vi "VisionMain_7.vi"(0 "Image In":T1, 7 "error in":errorcluster) -> (20 "Image Out":T1, 21 "Calibrated Centroid (PegLocation)":cluster{"X Centroid":sgl, "Y Centroid":sgl} {"Y Centroid" format="%.2f"; "X Centroid" format="%.2f"}, 22 "Particle Measurements (Real-World) (BoxValues)":dbl[][](array[numeric]) format="%.2f", 27 "error out":errorcluster)   [LabVIEW 2016]
uses:
  <vilib>/vision/Image Controls.llb/IMAQ Image.ctl
  <vilib>/vision/NI_Vision_Development_Module.lvlib
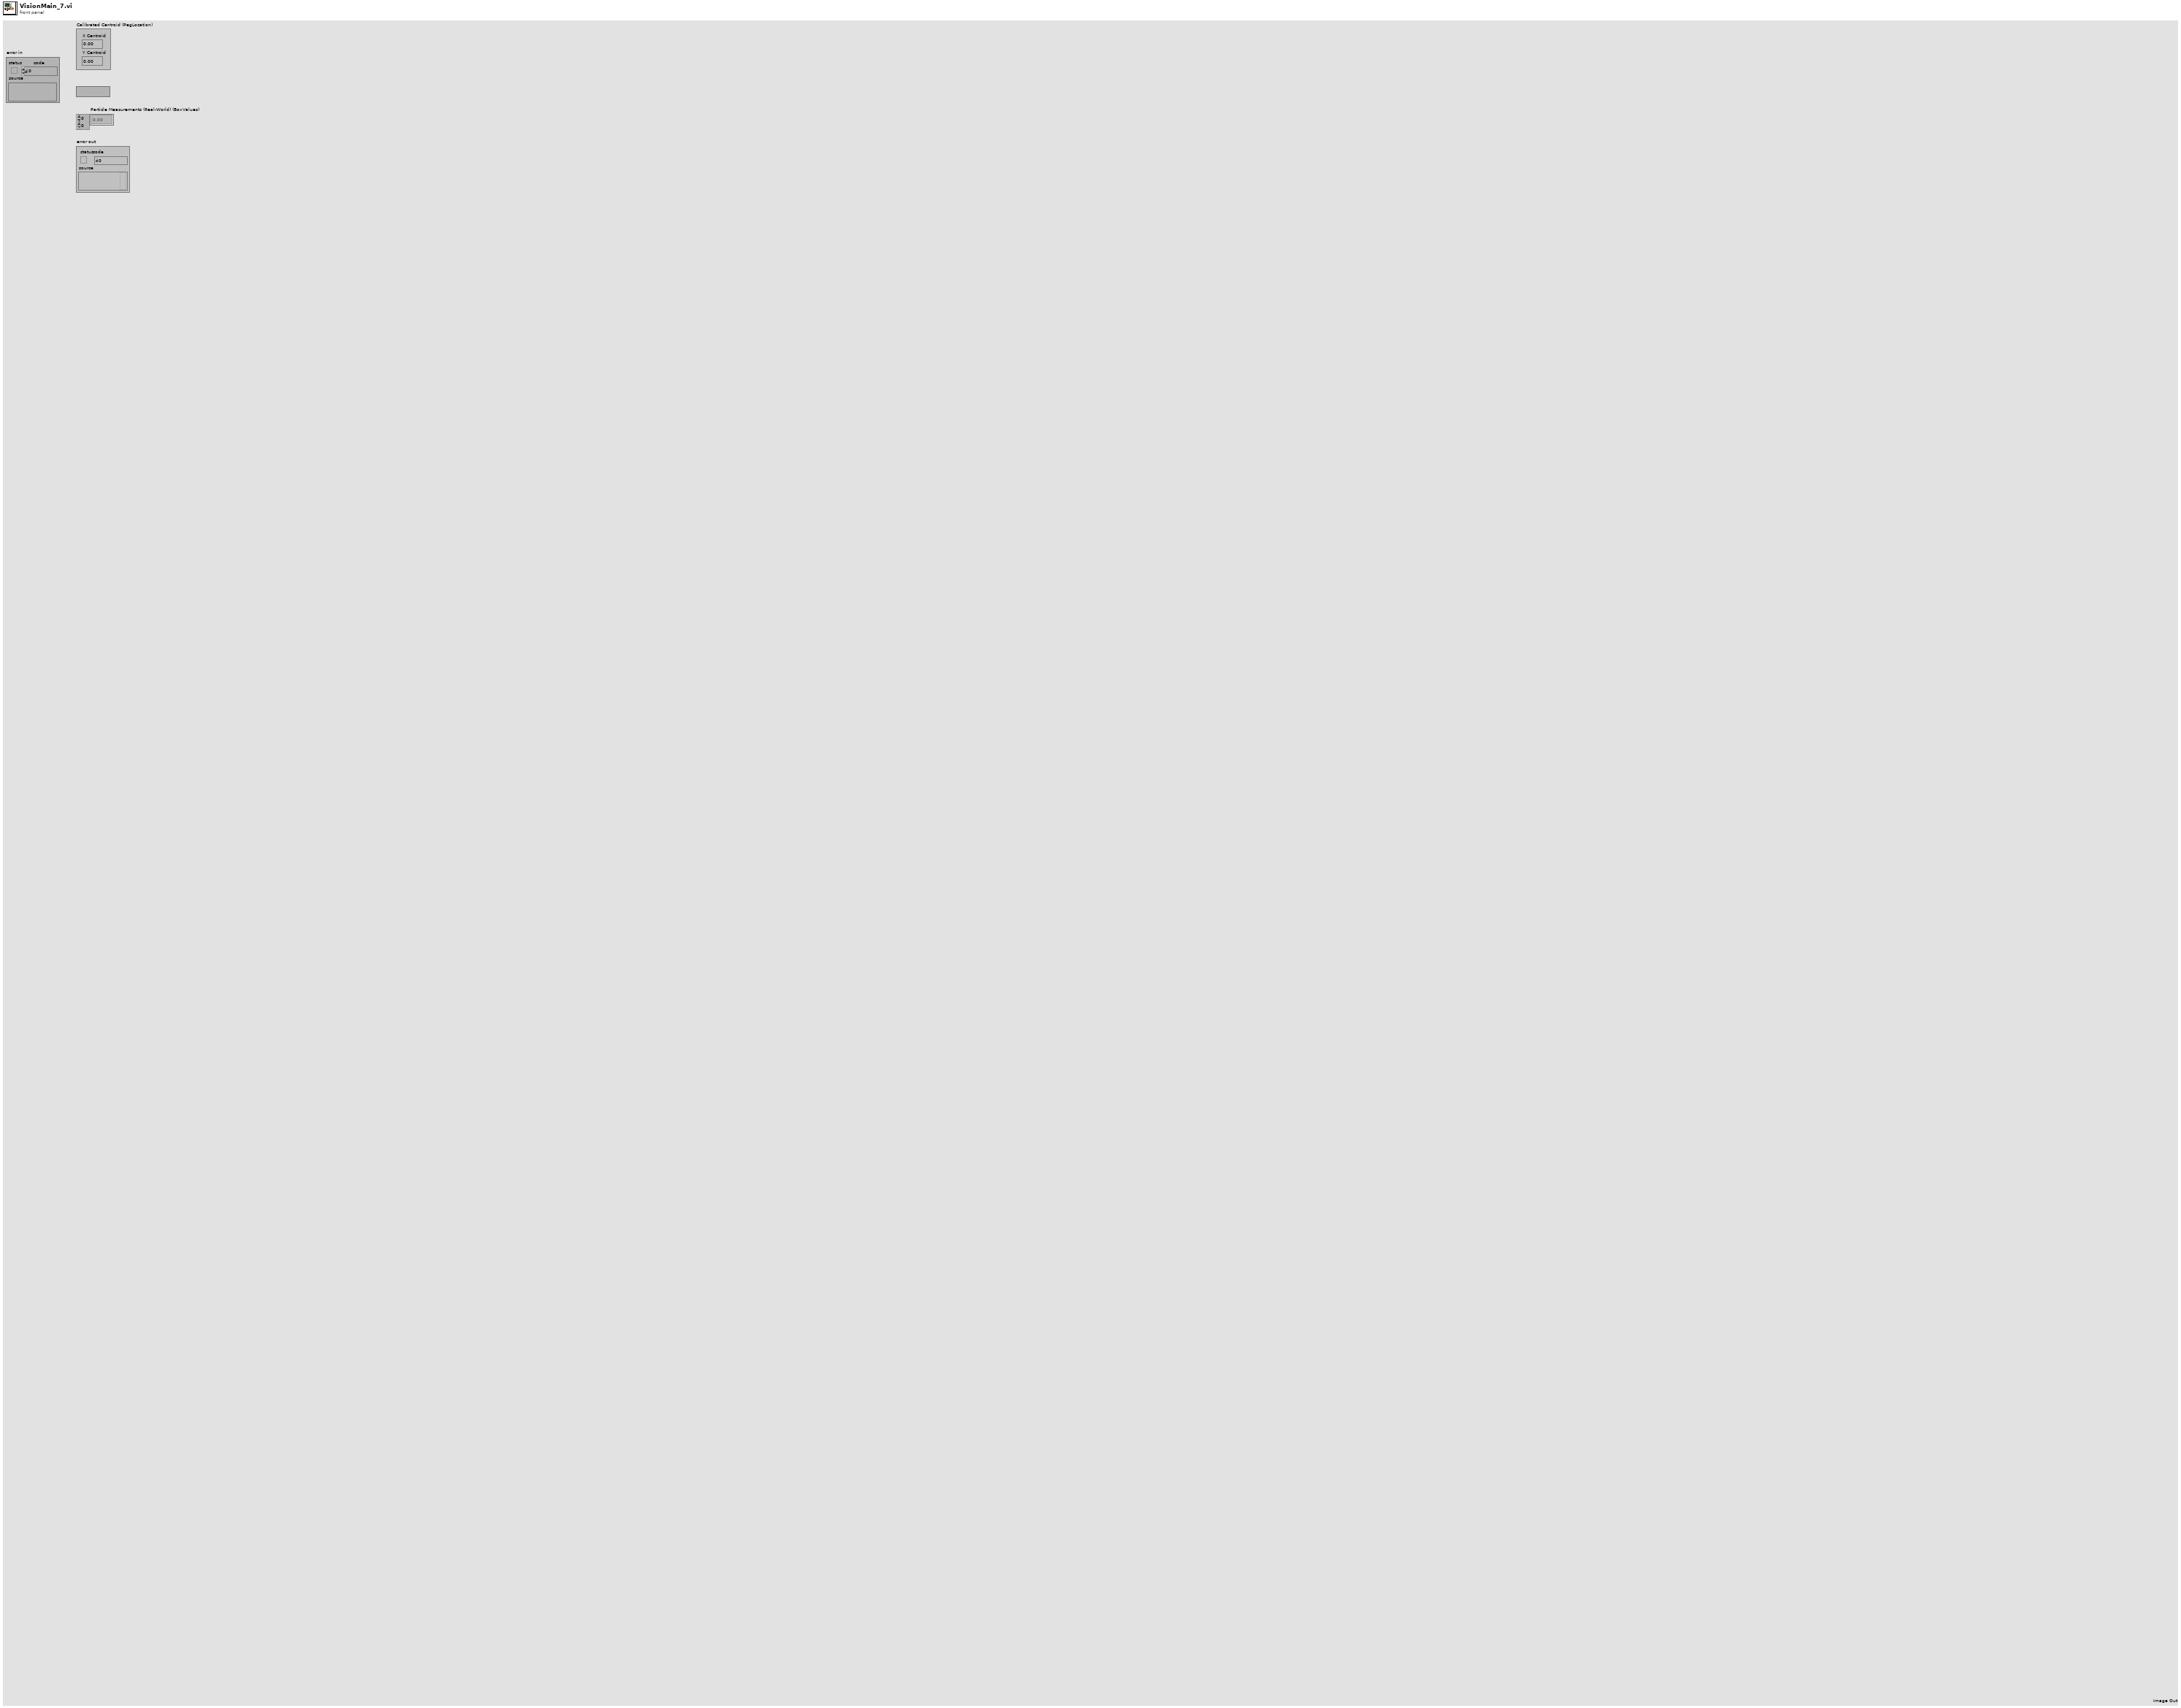
[diagram p1: front panel]
types:
  T1 = typedef "IMAQ Image.ctl" = refnum<image>
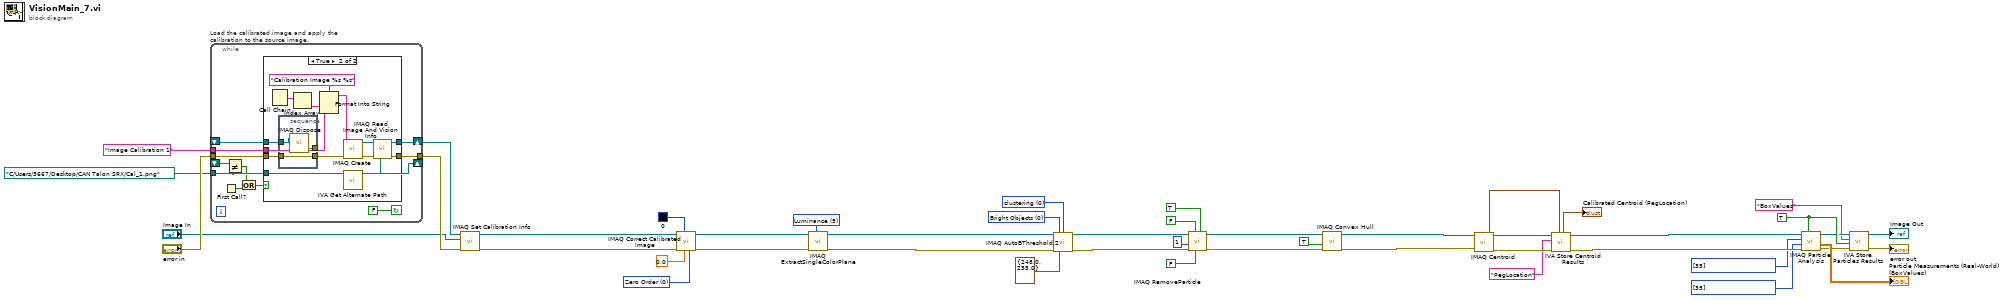
[diagram p0: block diagram]
diagram:
  w9 = i32[] [35] items=["Center of Mass X", "Center of Mass Y", "First Pixel X", "First Pixel Y", "Bounding Rect Left", "Bounding Rect Top", "Bounding Rect Right", "Bounding Rect Bottom", "Max Feret Diameter Start X", "Max Feret Diameter Start Y", "Max Feret Diameter End X", "Max Feret Diameter End Y", "Max Horiz. Segment Length Left", "Max Horiz. Segment Length Right", "Max Horiz. Segment Length Row", "-", "Bounding Rect Width", "Bounding Rect Height", "Bounding Rect Diagonal", "Perimeter", "Convex Hull Perimeter", "Holes' Perimeter", "Max Feret Diameter", "Equivalent Ellipse Major Axis", "Equivalent Ellipse Minor Axis", "Equivalent Ellipse Minor Axis (Feret)", "Equivalent Rect Long Side", "Equivalent Rect Short Side", "Equivalent Rect Diagonal", "Equivalent Rect Short Side (Feret)", "Average Horiz. Segment Length", "Average Vert. Segment Length", "Hydraulic Radius", "Waddel Disk Diameter", "-", "Area", "Holes' Area", "Particle & Holes' Area", "Convex Hull Area", "Image Area", "-", "Number of Holes", "Number of Horiz. Segments", "Number of Vert. Segments", "-", "Orientation", "Max Feret Diameter Orientation", "-", "% Area/Image Area", "% Area/(Particle & Holes' Area)", "Ratio of Equivalent Ellipse Axes", "Ratio of Equivalent Rect Sides", "-", "Elongation Factor", "Compactness Factor", "Heywood Circularity Factor", "Type Factor", "-", "Sum X", "Sum Y", "Sum XX", "Sum XY", "Sum YY", "Sum XXX", "Sum XXY", "Sum XYY", "Sum YYY", "-", "Moment of Inertia XX", "Moment of Inertia XY", "Moment of Inertia YY", "Moment of Inertia XXX", "Moment of Inertia XXY", "Moment of Inertia XYY", "Moment of Inertia YYY", "Norm. Moment of Inertia XX", "Norm. Moment of Inertia XY", "Norm. Moment of Inertia YY", "Norm. Moment of Inertia XXX", "Norm. Moment of Inertia XXY", "Norm. Moment of Inertia XYY", "Norm. Moment of Inertia YYY", "Hu Moment 1", "Hu Moment 2", "Hu Moment 3", "Hu Moment 4", "Hu Moment 5", "Hu Moment 6", "Hu Moment 7"] ("Real-World Measurements")
  w10 = i32[] [35] items=["Center of Mass X", "Center of Mass Y", "First Pixel X", "First Pixel Y", "Bounding Rect Left", "Bounding Rect Top", "Bounding Rect Right", "Bounding Rect Bottom", "Max Feret Diameter Start X", "Max Feret Diameter Start Y", "Max Feret Diameter End X", "Max Feret Diameter End Y", "Max Horiz. Segment Length Left", "Max Horiz. Segment Length Right", "Max Horiz. Segment Length Row", "-", "Bounding Rect Width", "Bounding Rect Height", "Bounding Rect Diagonal", "Perimeter", "Convex Hull Perimeter", "Holes' Perimeter", "Max Feret Diameter", "Equivalent Ellipse Major Axis", "Equivalent Ellipse Minor Axis", "Equivalent Ellipse Minor Axis (Feret)", "Equivalent Rect Long Side", "Equivalent Rect Short Side", "Equivalent Rect Diagonal", "Equivalent Rect Short Side (Feret)", "Average Horiz. Segment Length", "Average Vert. Segment Length", "Hydraulic Radius", "Waddel Disk Diameter", "-", "Area", "Holes' Area", "Particle & Holes' Area", "Convex Hull Area", "Image Area", "-", "Number of Holes", "Number of Horiz. Segments", "Number of Vert. Segments", "-", "Orientation", "Max Feret Diameter Orientation", "-", "% Area/Image Area", "% Area/(Particle & Holes' Area)", "Ratio of Equivalent Ellipse Axes", "Ratio of Equivalent Rect Sides", "-", "Elongation Factor", "Compactness Factor", "Heywood Circularity Factor", "Type Factor", "-", "Sum X", "Sum Y", "Sum XX", "Sum XY", "Sum YY", "Sum XXX", "Sum XXY", "Sum XYY", "Sum YYY", "-", "Moment of Inertia XX", "Moment of Inertia XY", "Moment of Inertia YY", "Moment of Inertia XXX", "Moment of Inertia XXY", "Moment of Inertia XYY", "Moment of Inertia YYY", "Norm. Moment of Inertia XX", "Norm. Moment of Inertia XY", "Norm. Moment of Inertia YY", "Norm. Moment of Inertia XXX", "Norm. Moment of Inertia XXY", "Norm. Moment of Inertia XYY", "Norm. Moment of Inertia YYY", "Hu Moment 1", "Hu Moment 2", "Hu Moment 3", "Hu Moment 4", "Hu Moment 5", "Hu Moment 6", "Hu Moment 7"] ("Pixel Measurements")
  w6 = TRUE ("Connectivity 4/8 (8)")
  w27 = 0 items=["clustering", "entropy", "metric", "moments", "inter-class variance"] ("Method")
  w28 = u32 0 items=["Bright Objects", "Dark Objects"] ("Look For")
  w33 = 5 items=["Red", "Green", "Blue", "Hue", "Saturation", "Luminance", "Value", "Intensity"] ("Color Plane")
  w38 = u32 0 items=["Zero Order", "Bi-Linear", "Quadratic", "Cubic Spline"] ("Interpolation Type")
  n1 = while "Load the calibrated image and apply the calibration to the source image." {
    shift-right: [w56] -> w43
    shift-left: _ -> [w55]
    tunnel: [w53] -> w42
    tunnel: "error in" -> [w52]
    tunnel: path "C:/Users/3667/Desktop/CAN Talon SRX/Cal_1.png" ("File Path") -> [w49]
    tunnel: "Image Calibration 1" ("Step Name") -> [w51]
    shift-right: [w49] -> _
    shift-left: _ -> [w50]
    stop <- FALSE continue-if-true
    n2 = First Call?() -> (First Call?: T/F=w48:bool)
    n3 = Not Equal?(x=w50, y=w49) -> (x != y?=w47:bool)
    n4 = Or(x=w47, y=w48) -> (x .or. y?=w46:bool)
    n5 = case shown="True" w46 {
      tunnel: [w58 w70] -> w56
      tunnel: w55 -> [w58 w62]
      tunnel: [w57 w67] -> w53
      tunnel: w52 -> [w57 w63]
      tunnel: w49 -> [_ w60]
      tunnel: w51 -> [_ w64]
      frame False {
      }
      frame True {
        n6 = Call Chain() -> (call chain=w66:string[])
        n7 = stacked-sequence {
          tunnel: w63 -> [w74]
          tunnel: w62 -> [w75]
          tunnel: [w74] -> w61
          tunnel: [w73] -> _
          frame #0 {
            n8 = call "IMAQ Dispose"("Image"=w75) -> ("error out"=w73:errorcluster)  [unwired: 2 in, 3 out]
          }
        }
        n9 = Index Array(array=w66) -> (element=w65:string)  [unwired: 1 in]
        n10 = Format Into String(format string="Calibration Image %s %s" ("Image Name"), w65, w64) -> (resulting string=w72:string)  [unwired: 2 in, 1 out]
        n11 = call "IMAQ Create"("Image Name"=w72, "error in (no error)"=w61) -> ("New Image"=w69:T1, "error out"=w68:errorcluster)  [unwired: 2 in, 1 out]
        n12 = call <vilib>:"IVA Get Alternate Path.vi"("Path In"=w60) -> ("Path Out"=w59:path)  [unwired: 10 out]
        n13 = call "IMAQ Read Image And Vision Info"("File Path"=w59, "error in (no error)"=w68, "Image"=w69) -> ("error out"=w67:errorcluster, "Image Out"=w70:T1)  [unwired: 1 in, 6 out]
      }
    }
  }
  n14 = call "IMAQ Set Calibration Info"("error in (no error)"=w42, "Image Dst"="Image In", "Image Src"=w43) -> ("error out"=w41:errorcluster, "Calibrated Image"=w36:T1)  [unwired: 1 in, 6 out]
  n15 = call "IMAQ Correct Calibrated Image"("Interpolation Type"=w38, "Replace Value"=sgl 0.0, "Color Replace Value"=u32 0, "error in (no error)"=w41, "Image Src"=w36) -> ("error out"=w37:errorcluster, "Corrected Image"=w32:T1)  [unwired: 2 in, 3 out]
  n16 = call "IMAQ ExtractSingleColorPlane"("Color Plane"=w33, "error in (no error)"=w37, "Image Src"=w32) -> ("error out"=w31:errorcluster, "Image Dst Out"=w30:T1)  [unwired: 1 in, 6 out]
  n17 = call "IMAQ AutoBThreshold 2"("Image Src"=w30, "Look For (Bright Objects)"=w28, "Method (clustering)"=w27, "error in (no error)"=w31, "Threshold Limits"=cluster{"Lower value":sgl, "Upper value":sgl} {"Lower value"=248.0, "Upper value"=255.0}) -> ("Image Dst Out"=w21:T1, "error out"=w29:errorcluster)  [unwired: 3 in, 6 out]
  n18 = call "IMAQ RemoveParticle"("Connectivity 4/8 (8)"=TRUE, "Low Pass/High Pass (Low)"=FALSE, "Square/Hexa (Square)"=FALSE, "error in (no error)"=w29, "Number of Erosion"=1, "Image Src"=w21) -> ("error out"=w20:errorcluster, "Image Dst Out"=w19:T1)  [unwired: 1 in, 3 out]
  n19 = call "IMAQ Convex Hull"("error in (no error)"=w20, "Connectivity 4/8 (8)"=TRUE, "Image Src"=w19) -> ("error out"=w17:errorcluster, "Image Dst Out"=w14:T1)  [unwired: 1 in, 6 out]
  n20 = call "IMAQ Centroid"("error in (no error)"=w17, "Image"=w14) -> ("error out"=w16:errorcluster, "Centroid"=w12:cluster{"X Centroid":sgl, "Y Centroid":sgl})  [unwired: 1 in, 1 out]
  n21 = call <vilib>:"IVA Store Centroid Results.vi"("Centroid in"=w12, "error in (no error)"=w16, "Step Name"="PegLocation", "Image in"=w14) -> ("error out"=w15:errorcluster, "Image dup"=w7:T1, "Calibrated Centroid"=→"Calibrated Centroid (PegLocation)":cluster{"X":sgl, "Y":sgl})  [unwired: 5 out]
  n22 = call "IMAQ Particle Analysis"("Connectivity 4/8 (8)"=w6, "error in (no error)"=w15, "Real-World Measurements"=w9, "Pixel Measurements"=w10, "Image"=w7) -> ("error out"=w2:errorcluster, "Particle Measurements (Real-World)"=→"Particle Measurements (Real-World) (BoxValues)":dbl[][], "Image Out (duplicate)"=w5:T1)  [unwired: 4 out]
  n23 = call <vilib>:"IVA Store Particles Results.vi"("error in (no error)"=w2, "Connectivity 4/8 (8)"=w6, "Step Name"="BoxValues", "Image in"=w5) -> ("error out"=→"error out":errorcluster, "Image dup"=→"Image Out":T1)  [unwired: 6 out]
